vi "TickstoHz.vi"(11 "Ticks":T1={"Low Ticks"=37, "High Ticks"=13}) -> (2 "Duty Cycle":dbl, 3 "Frequency":dbl)   [LabVIEW 2013, in "PWM Engine.lvlib"]
uses:
  PWM Engine.lvlib
  Shared/Types/PWM.ctl
  Shared/PWM Shared.lvlib
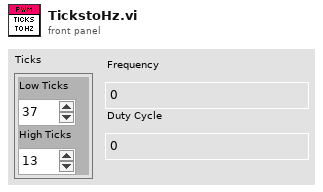
[diagram p1: front panel]
types:
  T1 = typedef "PWM Shared.lvlib/PWM.ctl" = cluster{"Low Ticks":u32, "High Ticks":u32}
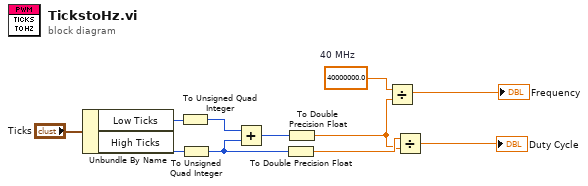
[diagram p0: block diagram]
diagram:
  w10 = 40000000.0  # 40 MHz
  n1 = Unbundle By Name("Ticks") -> ("Low Ticks"=w2:u32, "High Ticks"=w1:u32)
  n2 = To Unsigned Quad Integer(1:w2) -> (0:w11:u64)
  n3 = To Unsigned Quad Integer(1:w1) -> (0:w7:u64)
  n4 = Add(x=w11, y=w7) -> (x+y=w9:u64)
  n5 = To Double Precision Float(number=w7) -> (double precision float=w6:dbl)
  n6 = To Double Precision Float(number=w9) -> (double precision float=w5:dbl)
  n7 = Divide(x=w10, y=w5) -> (x/y=→"Frequency":dbl)
  n8 = Divide(x=w6, y=w5) -> (x/y=→"Duty Cycle":dbl)
